vi "InitializeDevice.vi"(8 "error in (no error)":errorcluster, 11 "NiPxi6123 in":refnum<class "NiPxi6123.lvclass">) -> (0 "error out":errorcluster, 3 "NiPxi6123 out":refnum<class "NiPxi6123.lvclass">)   [LabVIEW 2014, in "SamplerPlugins.lvlib" / "NiPxi6123.lvclass"]
uses:
  NiPxi6123.lvclass
  <vilib>/DAQmx/create/channels.llb/DAQmx Create Channel (AI-Voltage-Basic).vi
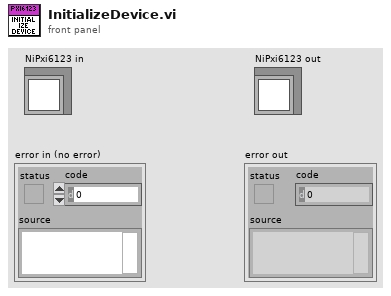
[diagram p1: front panel]
types:
  T1 = typedef "sPhysicalChannels.ctl" = string[]
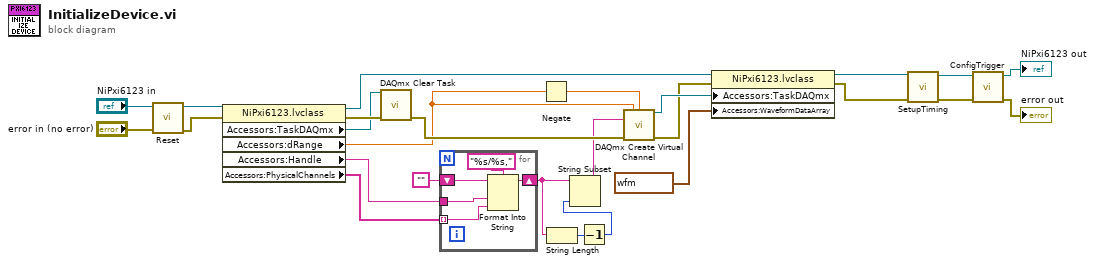
[diagram p0: block diagram]
diagram:
  n1 = call-dynamic "Reset.vi"("error in (no error)"="error in (no error)", "NiPxi6123 in"="NiPxi6123 in") -> ("error out"=w10:errorcluster, "NiPxi6123 out"=w11:refnum<class "NiPxi6123.lvclass">)  [unwired: 8 in]
  n2 = property class="NiPxi6123.lvclass"(reference=w11, error in=w10) -> (reference out=w12:refnum<class "NiPxi6123.lvclass">, error out=w16:errorcluster, "Accessors:TaskDAQmx"=w14:refnum<k21>, "Accessors:dRange"=w13:dbl, "Accessors:Handle"=w8:string, "Accessors:PhysicalChannels"=w7:T1)
  n3 = call <vilib>:"DAQmx Clear Task.vi"("task in"=w14, "error in"=w16) -> ("error out"=w15:errorcluster)  [unwired: 13 in]
  n4 = for {
    tunnel: w8 -> [w29]
    tunnel: w7 -> [w28] mode=indexing
    shift-right: [w27] -> w5
    shift-left: "" -> [w31]
    n5 = Format Into String(format string="%s/%s,", initial string=w31, w29, w28) -> (resulting string=w27:string)  [unwired: 1 in, 1 out]
  }
  n6 = Negate(x=w13) -> (-x=w17:dbl)
  n7 = String Length(string=w5) -> (length=w4:i32)
  n8 = Decrement(x=w4) -> (x-1=w3:i32)
  n9 = String Subset(string=w5, length (rest)=w3) -> (substring=w2:string)  [unwired: 1 in]
  n10 = call-poly <vilib>:"DAQmx Create Virtual Channel.vi"("maximum value"=w13, "minimum value"=w17, "physical channels"=w2, "error in"=w15) -> ("task out"=w9:refnum<k21>, "error out"=w1:errorcluster)  [unwired: 10 in]
  n11 = property class="NiPxi6123.lvclass"(reference=w12, error in=w1, "Accessors:TaskDAQmx"=w9, "Accessors:WaveformDataArray"=waveform(dbl)[] [{"t0"=timestamp(0 s since 1904-01-01), "dt"=1.0, "Y"=[0.0, 0.0, 0.0, 0.0, 0.0, 0.0, 0.0, 0.0, 0.0]}, {"t0"=timestamp(0 s since 1904-01-01), "dt"=1.0, "Y"=[0.0, 0.0, 0.0, 0.0, 0.0, 0.0, 0.0, 0.0, 0.0]}, {"t0"=timestamp(0 s since 1904-01-01), "dt"=1.0, "Y"=[0.0, 0.0, 0.0, 0.0, 0.0, 0.0, 0.0, 0.0, 0.0]}, {"t0"=timestamp(0 s since 1904-01-01), "dt"=1.0, "Y"=[0.0, 0.0, 0.0, 0.0, 0.0, 0.0, 0.0, 0.0, 0.0]}, {"t0"=timestamp(0 s since 1904-01-01), "dt"=1.0, "Y"=[0.0, 0.0, 0.0, 0.0, 0.0, 0.0, 0.0, 0.0, 0.0]}, {"t0"=timestamp(0 s since 1904-01-01), "dt"=1.0, "Y"=[0.0, 0.0, 0.0, 0.0, 0.0, 0.0, 0.0, 0.0, 0.0]}, {"t0"=timestamp(0 s since 1904-01-01), "dt"=1.0, "Y"=[0.0, 0.0, 0.0, 0.0, 0.0, 0.0, 0.0, 0.0, 0.0]}, {"t0"=timestamp(0 s since 1904-01-01), "dt"=1.0, "Y"=[0.0, 0.0, 0.0, 0.0, 0.0, 0.0, 0.0, 0.0, 0.0]}] ("WaveformDataArray")) -> (reference out=w21:refnum<class "NiPxi6123.lvclass">, error out=w20:errorcluster)
  n12 = call "SetupTiming.vi"("error in (no error)"=w20, "ClassIn"=w21) -> ("error out"=w23:errorcluster, "ClassOut"=w22:refnum<class "NiPxi6123.lvclass">)  [unwired: 8 in]
  n13 = call-dynamic "ConfigTrigger.vi"("error in (no error)"=w23, "NiPxi6123 in"=w22) -> ("error out"=→"error out":errorcluster, "NiPxi6123 out"=→"NiPxi6123 out":refnum<class "NiPxi6123.lvclass">)  [unwired: 8 in]
